vi "Read Operation Mode Status.vi"(8 "error in (no error)":errorcluster, 11 "Honeywell Compass HMC6343":refnum<class "Honeywell Compass HMC6343.lvclass">) -> (0 "error out":errorcluster, 1 "Operational Mode":u8(ring) items=["Standby Mode", "Run Mode"], 2 "Orientation":u8(ring) items=["Level Orientation", "Upright Edge Orientation", "Upright Front Orientation"], 3 "Honeywell Compass HMC6343 out":refnum<class "Honeywell Compass HMC6343.lvclass">, 4 "Calculating Calibration?":bool, 5 "Filter Used?":bool, 6 "Calculating Compass Data?":bool)   [LabVIEW 2019, in "Honeywell Compass HMC6343.lvclass"]
doc: "Reads the operation mode status of the device."
uses:
  Honeywell Compass HMC6343.lvclass
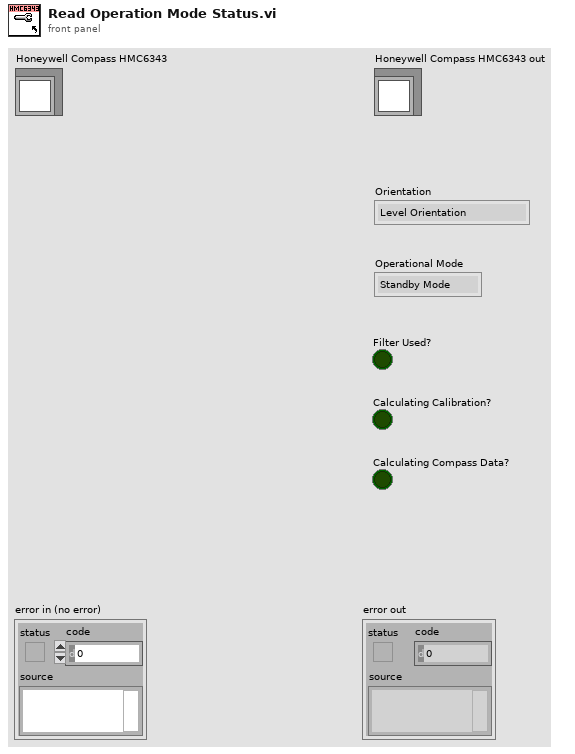
[diagram p1: front panel]
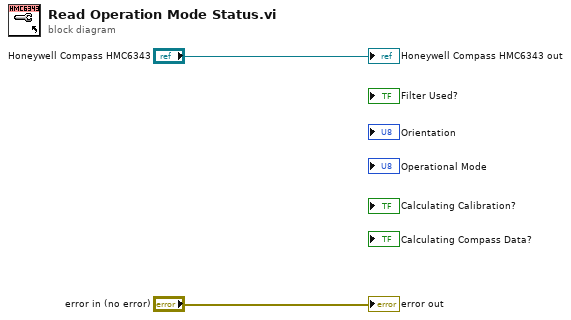
[diagram p0: block diagram]
diagram:
  "error out" <- "error in (no error)"
  "Honeywell Compass HMC6343 out" <- "Honeywell Compass HMC6343"
